vi "Read UI Constants.vi"(8 "error in":errorcluster, 11 "CFG File refnum in":T2) -> (0 "error out":errorcluster, 2 "output cluster":T1, 3 "CFG File refnum out":T2)   [LabVIEW 2015]
uses:
  <vilib>/Utility/config.llb/Config Data RefNum.ctl
  controls/MHL Configuration.ctl
  Boiler System Globals.vi
  <vilib>/Utility/config.llb/Read Key (Double).vi
  <vilib>/Utility/config.llb/NI_LVConfig.lvlib
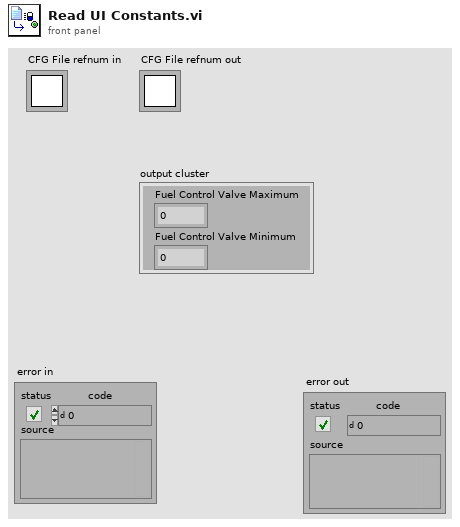
[diagram p1: front panel]
types:
  T1 = typedef "MHL Configuration.ctl" = cluster{"Fuel Control Valve Maximum":dbl, "Fuel Control Valve Minimum":dbl}
  T2 = typedef "NI_LVConfig.lvlib/Config Data RefNum.ctl" = refnum<k1>
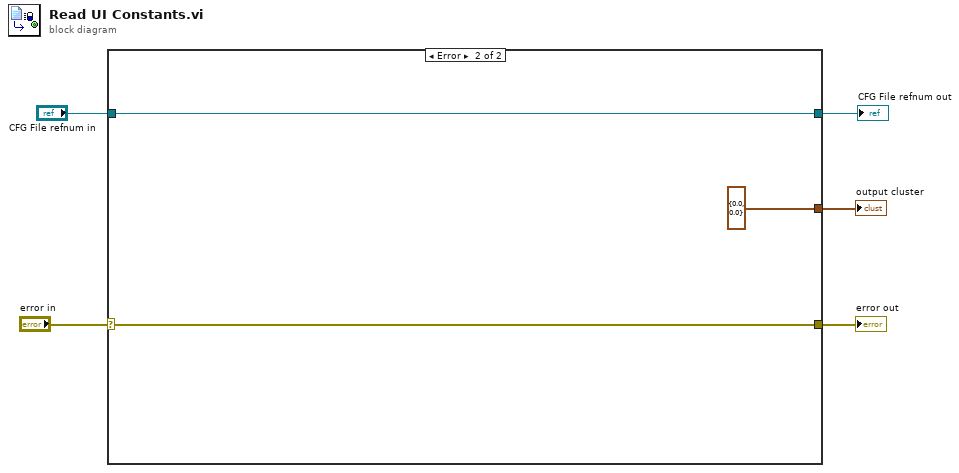
[diagram p0: block diagram]
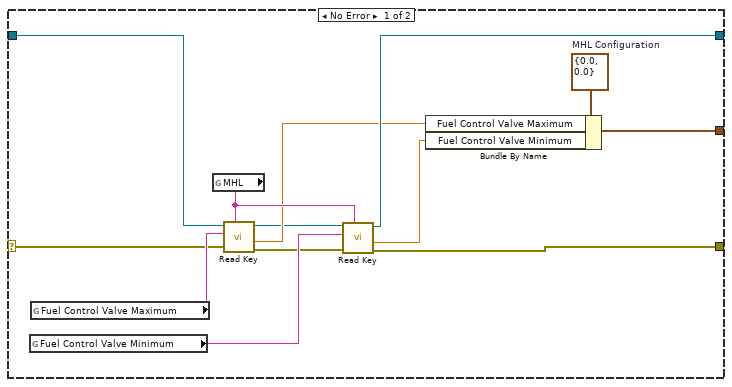
[diagram p2: hidden frame]
diagram:
  n1 = case shown="Error" "error in" {
    selector: "error in" -> [w14 w19]
    tunnel: "CFG File refnum in" -> [w17 w20]
    tunnel: [w12 w19] -> w3
    tunnel: [w11 w20] -> w2
    tunnel: [w7 T1 {"Fuel Control Valve Maximum"=0.0, "Fuel Control Valve Minimum"=0.0} ("MHL Configuration")] -> w1
    frame No Error {
      w10 = T1 {"Fuel Control Valve Maximum"=0.0, "Fuel Control Valve Minimum"=0.0}  # MHL Configuration
      n2 = global read "Boiler System Globals.vi" "Fuel Control Valve Minimum"() -> (w15:string)
      n3 = global read "Boiler System Globals.vi" "Fuel Control Valve Maximum"() -> (w16:string)
      n4 = global read "Boiler System Globals.vi" "MHL"() -> (w18:string)
      n5 = call-poly <vilib>:"Read Key.vi"("section"=w18, "error in (no error)"=w14, "key"=w16, "refnum"=w17) -> ("error out"=w13:errorcluster, "value"=w9:dbl, "refnum out"=w6:T2)  [unwired: 4 in, 1 out]
      n6 = call-poly <vilib>:"Read Key.vi"("section"=w18, "error in (no error)"=w13, "key"=w15, "refnum"=w6) -> ("error out"=w12:errorcluster, "value"=w8:dbl, "refnum out"=w11:T2)  [unwired: 4 in, 1 out]
      n7 = Bundle By Name(cluster=w10, "Fuel Control Valve Maximum"=w9, "Fuel Control Valve Minimum"=w8) -> (w7:T1)
    }
    frame Error {
    }
  }
  "error out" <- w3
  "CFG File refnum out" <- w2
  "output cluster" <- w1
